vi "tools_protoc.vi"() -> ()   [LabVIEW 2020]
uses:
  _subvis/Protoc UI State.ctl
  _subvis/Protoc UI Data.ctl
  LV-Proto/Enumeration.ctl
  LV-Proto/Enum Value.ctl
  LV-Proto/Message.ctl
  LV-Proto/Field.ctl
  LV-Proto/Type.ctl
  LV-Proto/Proto Type.ctl
  lv-userprefs/User Prefs/Pref Group/Pref Group.lvclass
  _subvis/Protoc UI Message.ctl
  _subvis/Protoc UI Command.ctl
  LV-Protoc/LV-Protoc/LV-Protoc.lvclass
  LV-Proto/LV-Proto.lvlib
  LV-Protoc/ProtoParser/ProtoParser.lvclass
  lv-userprefs/User Prefs/PrefsDB/PrefsDB.lvclass
  lv-cdm/CDM-Config/CDM-Config.lvlib
panel:
  out "Tab":T1(tab)
  in  "Begin":bool
  out ".proto Path":string
  in  "Include Paths":cluster{"Path":path, "Remove":bool}[](array[cluster])
  in  "Add Include":bool
  in  "Parse":bool
  in  "Cancel Parse":bool
  out "Messages":i32(listbox)
  out "Enumerations":i32(listbox)
  in  "Cancel Build":bool
  in  "Build":bool
  in  "Reset":bool
  # "This tool will walk you through selecting a .proto file to build LabVIEW code from along with configuring the code generation options.\n\nOnce complete, the new code will be displayed in an unsaved project to easily be moved into other projects or the new project can be saved."
  # "Add additional include paths for proto definitions."
  # "Parsing .proto files, please wait..."
  # "Review the following and continue to Build"
  # "You will select the output folder once you click Build."
  # "Generating LabVIEW code, please wait..."
  # "Generation has completed, review the generated project to see the generated code.\n\nYou may now close the tool or reset to process another .proto file."
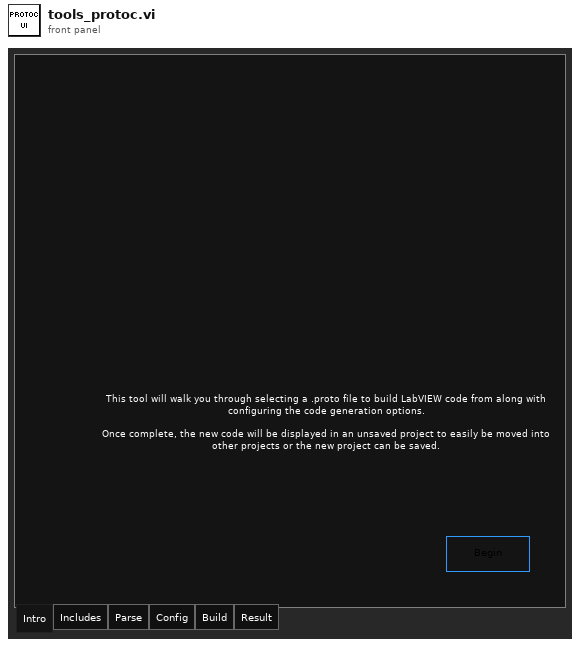
[diagram p1: front panel]
types:
  T1 = enum32{"Intro", "Includes", "Parse", "Config", "Build", "Result"}
  T2 = typedef "Protoc UI Message.ctl" = cluster{"Command":T3, "Data":variant}
  T3 = typedef "Protoc UI Command.ctl" = enum16{"Close", "Begin", "Parse", "Build", "Cancel"}
  T4 = typedef "Protoc UI Data.ctl" = cluster{".proto Path":path, "Enumerations":map{string, T5}, "Messages":map{string, T7}, "Include Paths":path[], "Output Folder":path, "Prefs":refnum<class "Pref Group.lvclass">}
  T5 = typedef "LV-Proto.lvlib/Enumeration.ctl" = cluster{"Name":string, "Values":T6[], "Reserved Numbers":u32[], "Reserved Names":string[]}
  T6 = typedef "LV-Proto.lvlib/Enum Value.ctl" = cluster{"Name":string, "Value":i32}
  T7 = typedef "LV-Proto.lvlib/Message.ctl" = cluster{"Name":string, "Fields":T8[], "Reserved Numbers":u32[], "Reserved Names":string[]}
  T8 = typedef "LV-Proto.lvlib/Field.ctl" = cluster{"Name":string, "Number":u32, "Optional":bool, "Repeated":bool, "Type":T9, "Key Type":T9, "Value Type":T9}
  T9 = typedef "LV-Proto.lvlib/Type.ctl" = cluster{"Type":T10, "Subtype":string}
  T10 = typedef "LV-Proto.lvlib/Proto Type.ctl" = enum16{"UNKNOWN", "double", "float", "int32", "int64", "uint32", "uint64", "sint32", "sint64", "fixed32", "fixed64", "sfixed32", "sfixed64", "bool", "string", "bytes", "enum", "map", "message"}
  T11 = typedef "Protoc UI State.ctl" = enum16{"Init", "Idle", "Select", "Includes", "Parse", "Options", "Build", "Complete"}
  T12 = cluster{"Shift":bool, "Ctrl":bool, "Alt":bool, "Cmd":bool, "Opt":bool}
  T13 = cluster{"Protoc UI Command":T3, "Variant":variant}
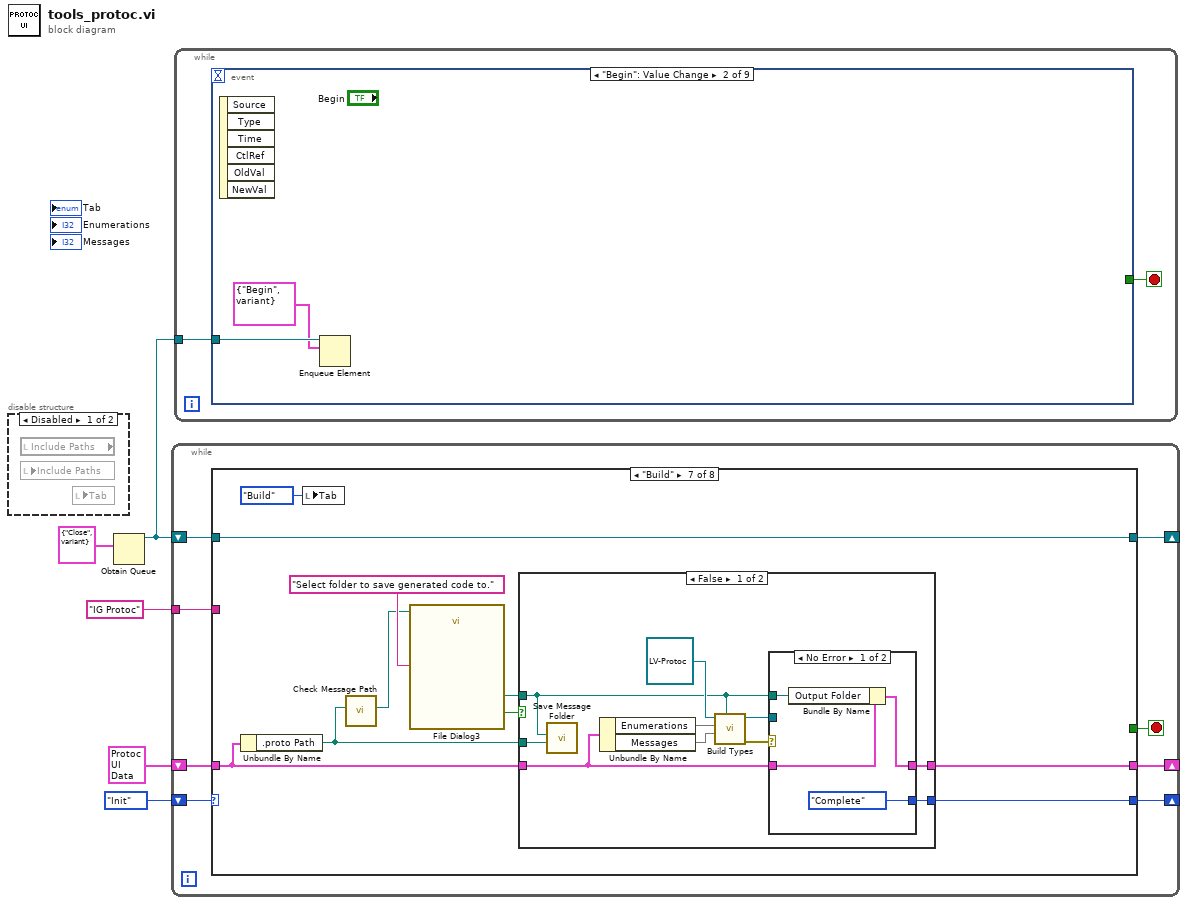
[diagram p0: block diagram]
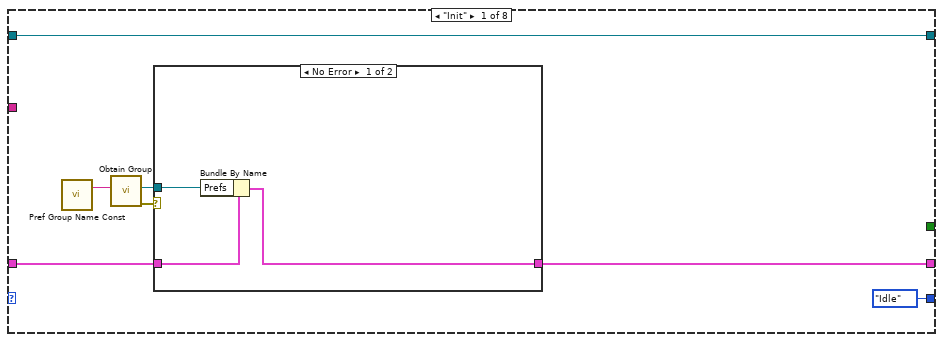
[diagram p3: hidden frame]
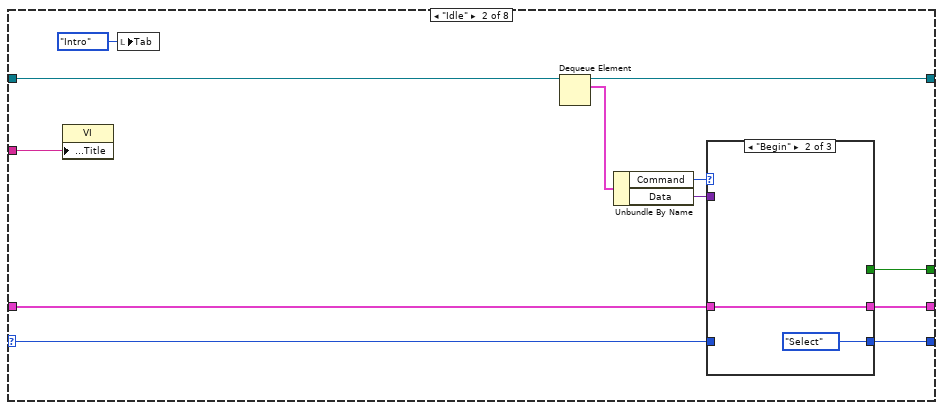
[diagram p5: hidden frame]
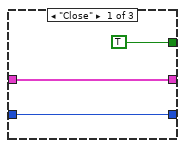
[diagram p6: hidden frame]
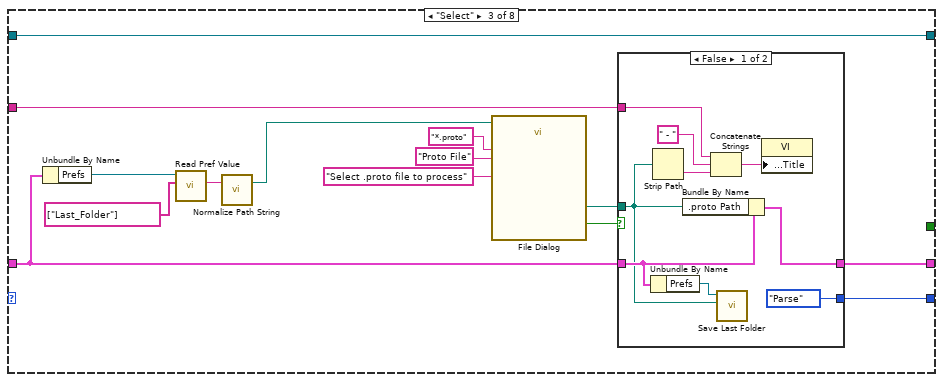
[diagram p8: hidden frame]
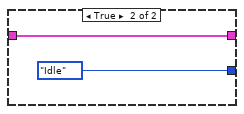
[diagram p9: hidden frame]
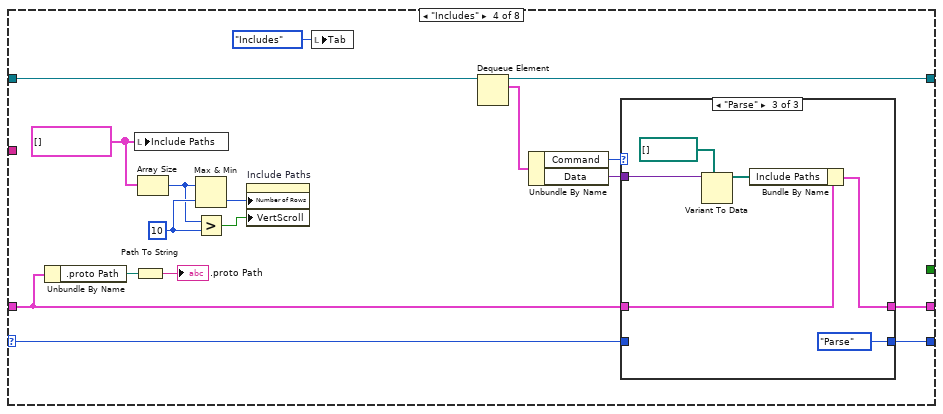
[diagram p10: hidden frame]
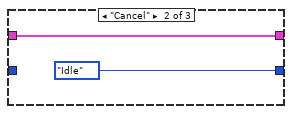
[diagram p12: hidden frame]
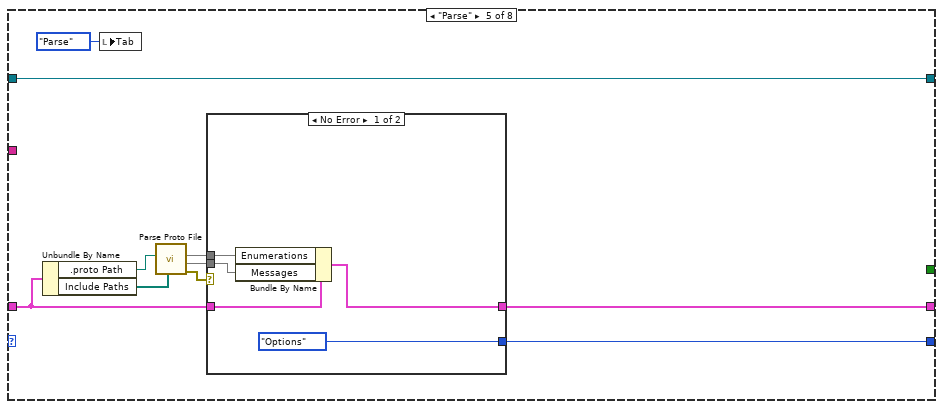
[diagram p13: hidden frame]
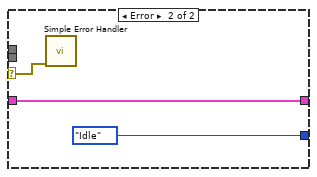
[diagram p14: hidden frame]
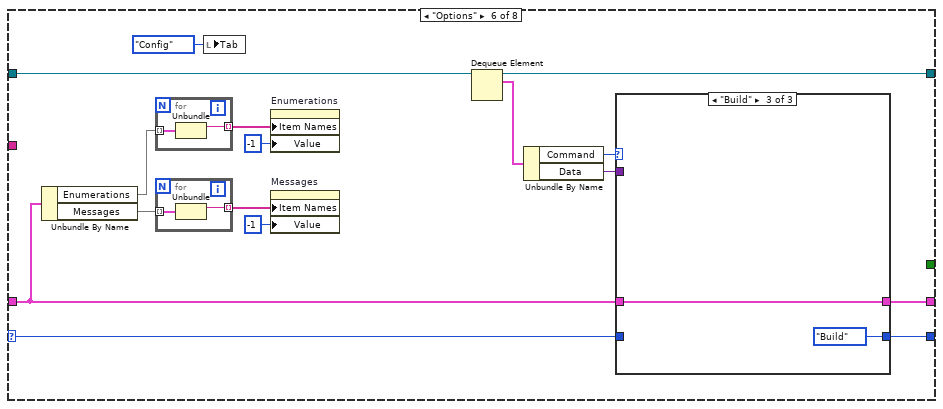
[diagram p15: hidden frame]
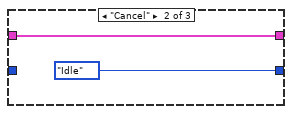
[diagram p17: hidden frame]
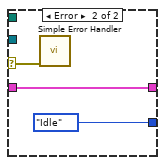
[diagram p18: hidden frame]
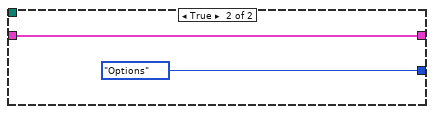
[diagram p19: hidden frame]
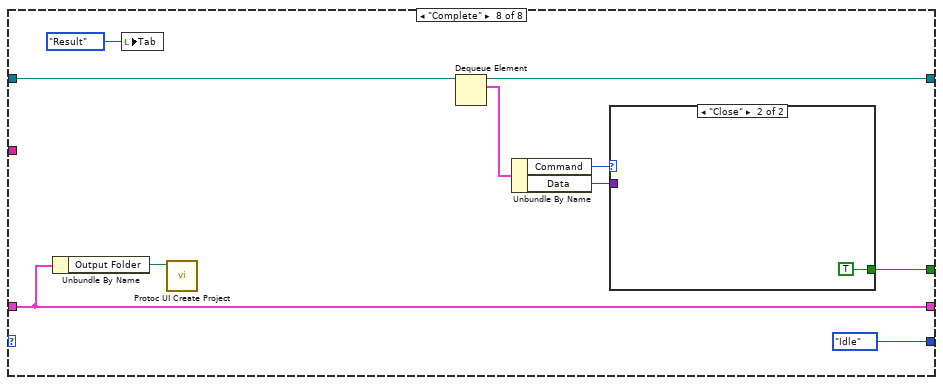
[diagram p20: hidden frame]
diagram:
  n1 = disable-structure shown="Disabled" {
    frame Disabled {
      n2 = local read "Include Paths"() -> ()  [unwired: 1 out]
      n3 = local read "Include Paths"() -> ()  [unwired: 1 in]
      n4 = local read "Tab"() -> ()  [unwired: 1 in]
    }
    frame Enabled {
    }
  }
  n5 = Obtain Queue(element data type=T2 {"Command"=enum."Close", "Data"=variant} ("Protoc UI Message")) -> (queue out=w2:refnum<queue>)  [unwired: 4 in, 2 out]
  n6 = while {
    shift-right: [w7] -> _
    shift-left: Protoc_UI_State."Init" ("Protoc UI State") -> [w13]
    shift-right: [w11] -> _
    shift-left: T4 {".proto Path"=path "", "Enumerations"={}, "Messages"={}, "Include Paths"=[], "Output Folder"=path "", "Prefs"=refnum} ("Protoc UI Data") -> [w12]
    shift-right: [w9] -> _
    shift-left: w2 -> [w10]
    tunnel: "IG Protoc" -> [w6]
    stop <- w8 stop-if-true
    n7 = case shown="\"Build\"" w13 {
      selector: w13 -> [_ w29 _ w78 _ w121 _ _]
      tunnel: w12 -> [w18 w31 w48 w71 w103 w120 w142 w170]
      tunnel: [w17 w27 w52 w79 w99 w122 w145 w170] -> w11
      tunnel: w10 -> [w20 w36 w57 w85 w105 w129 w149 w178]
      tunnel: [w20 w35 w57 w84 w105 w127 w149 w177] -> w9
      tunnel: [_ w30 _ _ _ _ _ w172] -> w8
      tunnel: [Protoc_UI_State."Idle" ("Protoc UI State") w28 w49 w80 w98 w123 w144 Protoc_UI_State."Idle" ("Protoc UI State")] -> w7
      tunnel: w6 -> [_ w25 w50 _ _ _ _ _]
      frame "Init" {
        n8 = call "Pref Group Name Const.vi"() -> ("Pref Group Name"=w14:string)  [unwired: 7 in]
        n9 = call "Obtain Group.vi"("Group"=w14) -> ("error out"=w15:errorcluster, "Pref Group"=w16:refnum<class "Pref Group.lvclass">)  [unwired: 8 in, 1 out]
        n10 = case shown="No Error" w15 {
          tunnel: w18 -> [w23 w24]
          tunnel: [w22 w24] -> w17
          tunnel: w16 -> [w21 _]
          frame No Error {
            n11 = Bundle By Name(cluster=w23, "Prefs"=w21) -> (w22:T4)
          }
          frame Error {
          }
        }
      }
      frame "Idle" {
        n12 = property class="VI"("Front Panel.Title"=w25) -> ()  [unwired: 2 in, 2 out]
        n13 = local write "Tab"(T1."Intro" ("Tab")) -> ()
        n14 = Dequeue Element(queue=w36) -> (queue out=w35:refnum<queue>, element=w34:T2)  [unwired: 2 in, 2 out]
        n15 = Unbundle By Name(w34) -> ("Command"=w33:T3, "Data"=w32:variant)
        n16 = case shown="\"Begin\"" w33 {
          tunnel: w32 -> [_ _ _]
          tunnel: w31 -> [w37 w40 w42]
          tunnel: [TRUE _ _] -> w30
          tunnel: w29 -> [w38 _ w43]
          tunnel: [w38 Protoc_UI_State."Select" ("Protoc UI State") w43] -> w28
          tunnel: [w37 w40 w42] -> w27
          frame "Close" {
          }
          frame "Begin" {
          }
          frame Default {
          }
        }
      }
      frame "Select" {
        n17 = Unbundle By Name(w48) -> ("Prefs"=w47:refnum<class "Pref Group.lvclass">)
        n18 = call "Read Pref Value.vi"("Pref Hierarchy"=string[] ["Last_Folder"], "Pref Group in"=w47) -> ("Value"=w44:string)  [unwired: 7 in, 2 out]
        n19 = call "Normalize Path String.vi"("Path String"=w44) -> ("Path"=w45:path)  [unwired: 2 in]
        n20 = call "File Dialog"("start path"=w45, "prompt"="Select .proto file to process", "pattern (all files)"="*.proto", "pattern label"="Proto File") -> ("selected path"=w53:path, "cancelled"=w51:bool)  [unwired: 8 in, 2 out]
        n21 = case shown="False" w51 {
          tunnel: w53 -> [w58 _]
          tunnel: [w66 w67] -> w52
          tunnel: w48 -> [w60 w67]
          tunnel: w50 -> [w64 _]
          tunnel: [Protoc_UI_State."Parse" ("Protoc UI State") Protoc_UI_State."Idle" ("Protoc UI State")] -> w49
          frame False {
            n22 = Unbundle By Name(w60) -> ("Prefs"=w59:refnum<class "Pref Group.lvclass">)
            n23 = Strip Path(path=w58) -> (name=w62:string)  [unwired: 1 out]
            n24 = Bundle By Name(cluster=w60, ".proto Path"=w58) -> (w66:T4)
            n25 = Concatenate Strings(w64, " - " ("string"), w62) -> (w61:string)
            n26 = call "Save Last Folder.vi"(".proto Path"=w58, "Pref Group"=w59) -> ()  [unwired: 9 in, 1 out]
            n27 = property class="VI"("Front Panel.Title"=w61) -> ()  [unwired: 2 in, 2 out]
          }
          frame True {
          }
        }
      }
      frame "Includes" {
        w77 = 10 ("y")
        w73 = cluster{"Path":path, "Remove":bool}[] [] ("Include Paths")
        n28 = Unbundle By Name(w71) -> (".proto Path"=w70:path)
        n29 = local write "Include Paths"(w73) -> ()
        n30 = Path To String(path=w70) -> (string=→".proto Path":string)
        n31 = Array Size(array=w73) -> (size(s)=w74:i32)
        n32 = Max & Min(x=w74, y=w77) -> (min(x,y)=w75:i32)  [unwired: 1 out]
        n33 = Greater?(x=w74, y=w77) -> (0:w76:bool)
        n34 = property on="Include Paths" class="Arr"("Number of Rows"=w75, "VertScroll"=w76) -> ()  [unwired: 2 in, 2 out]
        n35 = local write "Tab"(T1."Includes" ("Tab")) -> ()
        n36 = Dequeue Element(queue=w85) -> (queue out=w84:refnum<queue>, element=w83:T2)  [unwired: 2 in, 2 out]
        n37 = Unbundle By Name(w83) -> ("Command"=w82:T3, "Data"=w81:variant)
        n38 = case shown="\"Parse\"" w82 {
          tunnel: w71 -> [w87 w88 w93]
          tunnel: w81 -> [_ _ w95]
          tunnel: [w86 Protoc_UI_State."Idle" ("Protoc UI State") Protoc_UI_State."Parse" ("Protoc UI State")] -> w80
          tunnel: [w87 w88 w91] -> w79
          tunnel: w78 -> [w86 _ _]
          frame Default {
          }
          frame "Cancel" {
          }
          frame "Parse" {
            n39 = Variant To Data(type=path[] [], Variant=w95) -> (data=w92:path[])  [unwired: 1 in, 1 out]
            n40 = Bundle By Name(cluster=w93, "Include Paths"=w92) -> (w91:T4)
          }
        }
      }
      frame "Parse" {
        n41 = Unbundle By Name(w103) -> (".proto Path"=w104:path, "Include Paths"=w97:path[])
        n42 = local write "Tab"(T1."Parse" ("Tab")) -> ()
        n43 = call "Parse Proto File.vi"("Include Paths (None)"=w97, ".proto Path"=w104) -> ("error out"=w102:errorcluster, "Messages"=w101:map{string, T7}, "Enumerations"=w100:map{string, T5})  [unwired: 6 in, 1 out]
        n44 = case shown="No Error" w102 {
          selector: w102 -> [_ w111]
          tunnel: w103 -> [w110 w113]
          tunnel: w101 -> [w108 _]
          tunnel: w100 -> [w109 _]
          tunnel: [w107 w113] -> w99
          tunnel: [Protoc_UI_State."Options" ("Protoc UI State") Protoc_UI_State."Idle" ("Protoc UI State")] -> w98
          frame No Error {
            n45 = Bundle By Name(cluster=w110, "Enumerations"=w109, "Messages"=w108) -> (w107:T4)
          }
          frame Error {
            n46 = call <vilib>:"Simple Error Handler.vi"("error in (no error)"=w111) -> ()  [unwired: 4 in, 5 out]
          }
        }
      }
      frame "Options" {
        n47 = Unbundle By Name(w120) -> ("Enumerations"=w119:map{string, T5}, "Messages"=w118:map{string, T7})
        n48 = for {
          tunnel: w119 -> [w133] mode=indexing
          tunnel: [w132] -> w117 mode=indexing
          n49 = Unbundle(w133) -> ("Name"=w132:string)  [unwired: 1 out]
        }
        n50 = for {
          tunnel: w118 -> [w131] mode=indexing
          tunnel: [w130] -> w116 mode=indexing
          n51 = Unbundle(w131) -> ("Name"=w130:string)  [unwired: 1 out]
        }
        n52 = local write "Tab"(T1."Config" ("Tab")) -> ()
        n53 = property on="Enumerations" class="LstBox (strict)"("Item Names"=w117, "Value"=-1 ("Enumerations")) -> ()  [unwired: 2 in, 2 out]
        n54 = property on="Messages" class="LstBox (strict)"("Item Names"=w116, "Value"=-1 ("Messages")) -> ()  [unwired: 2 in, 2 out]
        n55 = Dequeue Element(queue=w129) -> (queue out=w127:refnum<queue>, element=w124:T2)  [unwired: 2 in, 2 out]
        n56 = Unbundle By Name(w124) -> ("Command"=w126:T3, "Data"=w125:variant)
        n57 = case shown="\"Build\"" w126 {
          tunnel: w125 -> [_ _ _]
          tunnel: [w134 Protoc_UI_State."Idle" ("Protoc UI State") Protoc_UI_State."Build" ("Protoc UI State")] -> w123
          tunnel: [w135 w136 w138] -> w122
          tunnel: w120 -> [w135 w136 w138]
          tunnel: w121 -> [w134 _ _]
          frame Default {
          }
          frame "Cancel" {
          }
          frame "Build" {
          }
        }
      }
      frame "Build" {
        n58 = Unbundle By Name(w142) -> (".proto Path"=w140:path)
        n59 = local write "Tab"(T1."Build" ("Tab")) -> ()
        n60 = call "Check Message Path.vi"(".proto Path"=w140) -> ("Starting Folder"=w141:path)  [unwired: 9 in, 1 out]
        n61 = call "File Dialog3"("start path"=w141, "prompt"="Select folder to save generated code to.") -> ("selected path"=w146:path, "cancelled"=w147:bool)  [unwired: 10 in, 2 out]
        n62 = case shown="False" w147 {
          tunnel: w142 -> [w152 w168]
          tunnel: w146 -> [w150 _]
          tunnel: [w153 w168] -> w145
          tunnel: [w157 Protoc_UI_State."Options" ("Protoc UI State")] -> w144
          tunnel: w140 -> [w151 _]
          frame False {
            n63 = call "Save Message Folder.vi"(".proto Path"=w151, "Output Folder"=w150) -> ()  [unwired: 9 in, 1 out]
            n64 = Unbundle By Name(w152) -> ("Enumerations"=w159:map{string, T5}, "Messages"=w158:map{string, T7})
            n65 = call "Build Types.vi"("Output Folder"=w150, "Messages"=w158, "Enumerations"=w159, "LV-Protoc in"=refnum<class "LV-Protoc.lvclass"> refnum) -> ("error out"=w156:errorcluster, "LV-Protoc out"=w155:refnum<class "LV-Protoc.lvclass">)  [unwired: 6 in]
            n66 = case shown="No Error" w156 {
              selector: w156 -> [_ w164]
              tunnel: [Protoc_UI_State."Complete" ("Protoc UI State") Protoc_UI_State."Idle" ("Protoc UI State")] -> w157
              tunnel: w155 -> [_ _]
              tunnel: [w161 w165] -> w153
              tunnel: w152 -> [w162 w165]
              tunnel: w150 -> [w160 _]
              frame No Error {
                n67 = Bundle By Name(cluster=w162, "Output Folder"=w160) -> (w161:T4)
              }
              frame Error {
                n68 = call <vilib>:"Simple Error Handler.vi"("error in (no error)"=w164) -> ()  [unwired: 4 in, 5 out]
              }
            }
          }
          frame True {
          }
        }
      }
      frame "Complete" {
        n69 = Unbundle By Name(w170) -> ("Output Folder"=w169:path)
        n70 = local write "Tab"(T1."Result" ("Tab")) -> ()
        n71 = call "Protoc UI Create Project.vi"("Output Folder"=w169) -> ()  [unwired: 11 in]
        n72 = Dequeue Element(queue=w178) -> (queue out=w177:refnum<queue>, element=w175:T2)  [unwired: 2 in, 2 out]
        n73 = Unbundle By Name(w175) -> ("Command"=w174:T3, "Data"=w173:variant)
        n74 = case shown="\"Close\"" w174 {
          tunnel: w173 -> [_ _]
          tunnel: [_ TRUE] -> w172
          frame Default {
          }
          frame "Close" {
          }
        }
      }
    }
  }
  n75 = while {
    tunnel: w2 -> [w181]
    stop <- w180 stop-if-true
    n76 = event shown="[1] \"Begin\": Value Change" {
      selector: _ -> [_ _ _ _ _ _ _ _ _]
      dyn-events: _ -> [_ _ _ _ _ _ _ _ _]
      timeout: _ -> [_ _ _ _ _ _ _ _ _]
      tunnel: w181 -> [_ w183 _ _ _ w219 w224 _ w231]
      tunnel: [_ _ _ _ _ _ _ w225 _] -> w180
      event Timeout {
        n77 = event-data() -> ()  [unwired: 1 in, 1 out]
      }
      event "Begin": Value Change {
        n78 = event-data() -> ()  [unwired: 1 in, 6 out]
        n79 = Enqueue Element(queue=w183, element=T2 {"Command"=enum."Begin", "Data"=variant} ("Protoc UI Message")) -> ()  [unwired: 2 in, 3 out]
      }
      event "Tab": Mouse Down? {
        n80 = event-data() -> ("Button"=w189:u16, "PlatMods"=w190:T12)  [unwired: 1 in, 6 out]
        n81 = Unbundle By Name(w190) -> ("Ctrl"=w187:bool, "Alt"=w186:bool)
        n82 = Equal?(x=u16 2, y=w189) -> (x = y?=w185:bool)
        n83 = Compound Arithmetic op=AND(w185, w187, w186) -> (w184:bool)
        n84 = case shown="True" w184 {
          frame False {
          }
          frame True {
            n85 = property class="VI"("BDWin.Open"=TRUE ("Block Diagram Window:Open")) -> ()  [unwired: 2 in, 2 out]
          }
        }
        n86 = event-data("Discard?"=w184) -> ()  [unwired: 1 in, 1 out]
      }
      event "Add Include": Value Change {
        n87 = event-data() -> ()  [unwired: 1 in, 1 out]
        n88 = call "File Dialog2"("prompt"="Select folder to add to include paths") -> ("selected path"=w192:path, "cancelled"=w193:bool)  [unwired: 11 in, 2 out]
        n89 = case shown="False" w193 {
          tunnel: w192 -> [w203 _]
          frame False {
            w198 = 10 ("y")
            n90 = local read "Include Paths"() -> (w201:cluster{"Path":path, "Remove":bool}[])
            n91 = Bundle("selected path"=w203, FALSE) -> (w200:cluster{"selected path":path, bool})  [unwired: 1 in]
            n92 = Build Array (concatenate)(w201, w200) -> (w199:cluster{"selected path":path, "Remove":bool}[])
            n93 = local write "Include Paths"(w199) -> ()
            n94 = Array Size(array=w199) -> (size(s)=w197:i32)
            n95 = Max & Min(x=w197, y=w198) -> (min(x,y)=w196:i32)  [unwired: 1 out]
            n96 = Greater?(x=w197, y=w198) -> (0:w195:bool)
            n97 = property on="Include Paths" class="Arr"("Number of Rows"=w196, "VertScroll"=w195) -> ()  [unwired: 2 in, 2 out]
          }
          frame True {
          }
        }
      }
      event "Include Paths": Value Change {
        n98 = event-data() -> ("NewVal"=w207:cluster{"Path":path, "Remove":bool}[])  [unwired: 1 in]
        n99 = for {
          tunnel: w207 -> [w217] mode=indexing
          tunnel: [w216] -> w205
          tunnel: [w215] -> w206
          i -> [w216]
          stop <- w215 stop-if-true
          n100 = Unbundle(w217) -> ("Remove"=w215:bool)  [unwired: 1 out]
        }
        n101 = case shown="True" w206 {
          tunnel: w205 -> [_ w213]
          tunnel: "Include Paths" -> [_ w214]
          frame False {
          }
          frame True {
            w209 = 10 ("y")
            n102 = Delete From Array(array=w214, index=w213) -> (array with subset deleted=w208:cluster{"Path":path, "Remove":bool}[])  [unwired: 1 in, 1 out]
            n103 = local write "Include Paths"(w208) -> ()
            n104 = Array Size(array=w208) -> (size(s)=w212:i32)
            n105 = Max & Min(x=w212, y=w209) -> (min(x,y)=w211:i32)  [unwired: 1 out]
            n106 = Greater?(x=w212, y=w209) -> (0:w210:bool)
            n107 = property on="Include Paths" class="Arr"("Number of Rows"=w211, "VertScroll"=w210) -> ()  [unwired: 2 in, 2 out]
          }
        }
      }
      event "Parse": Value Change {
        n108 = event-data() -> ()  [unwired: 1 in, 1 out]
        n109 = local read "Include Paths"() -> (w222:cluster{"Path":path, "Remove":bool}[])
        n110 = To Variant(anything=w222) -> (Variant=w221:variant)
        n111 = Bundle("Protoc UI Command"=Protoc_UI_Command."Parse", "Variant"=w221) -> (w218:T13)  [unwired: 1 in]
        n112 = Enqueue Element(queue=w219, element=w218) -> ()  [unwired: 2 in, 3 out]
      }
      event "Build": Value Change {
        n113 = event-data() -> ()  [unwired: 1 in, 6 out]
        n114 = Enqueue Element(queue=w224, element=T2 {"Command"=enum."Build", "Data"=variant} ("Protoc UI Message")) -> ()  [unwired: 2 in, 3 out]
      }
      event Panel Close? {
        n115 = event-data() -> ()  [unwired: 1 in, 4 out]
        n116 = local read "Tab"() -> (w227:T1)
        n117 = case shown="Default" w227 {
          tunnel: [TRUE _] -> w226
          frame Default {
            n118 = One Button Dialog(message="The tool cannot be closed while the tool is running.\n\nCancel the configuration and then the tool can be closed.") -> ()  [unwired: 1 in, 1 out]
          }
          frame "Intro", "Result" {
          }
        }
        n119 = event-data("Discard?"=w226) -> ()  [unwired: 1 in, 1 out]
        n120 = Not(x=w226) -> (.not. x?=w225:bool)
      }
      event "Cancel Parse", "Cancel Build", "Reset": Value Change {
        n121 = event-data() -> ()  [unwired: 1 in, 1 out]
        n122 = Enqueue Element(queue=w231, element=T2 {"Command"=enum."Cancel", "Data"=variant} ("Protoc UI Message")) -> ()  [unwired: 2 in, 3 out]
      }
    }
  }
